vi "Get Channel Details.vi"(11 "Channel Parameters In":T1={"Channel Name"="0", "Number of Records"=0, "Reference Position"=0.0, "Minimum Record Length"=0, "Minimum Sample Rate"=0.0, "Maximum Input Frequency"=0.0, "Enforce Realtime"=FALSE, "Vertical Coupling"=enum."AC", "Probe Attenuation"=0.0, "Vertical Range (V)"=0.0, "Vertical Offset"=0.0, "Trigger Level"=0.0, "Trigger Type"=enum."Edge", "Trigger Source"=enum."Immediate", "Trigger Slope"=enum."Positive", "Digitizer 1 Used?"=FALSE, "Digitizer 1 Channels"="", "Digitizer 1 Reference"="", "Digitizer 1 Gain Multiplier"=nan, "Digitizer 2 Used?"=FALSE, "Digitizer 2 Channels"="", "Digitizer 2 Reference"="", "Session References"=[]}) -> (3 "Channel Parameters Out":T1={"Channel Name"="0", "Number of Records"=0, "Reference Position"=0.0, "Minimum Record Length"=0, "Minimum Sample Rate"=0.0, "Maximum Input Frequency"=0.0, "Enforce Realtime"=FALSE, "Vertical Coupling"=enum."AC", "Probe Attenuation"=0.0, "Vertical Range (V)"=0.0, "Vertical Offset"=0.0, "Trigger Level"=0.0, "Trigger Type"=enum."Edge", "Trigger Source"=enum."Immediate", "Trigger Slope"=enum."Positive", "Digitizer 1 Used?"=FALSE, "Digitizer 1 Channels"="", "Digitizer 1 Reference"="", "Digitizer 1 Gain Multiplier"=nan, "Digitizer 2 Used?"=FALSE, "Digitizer 2 Channels"="", "Digitizer 2 Reference"="", "Session References"=[]})   [LabVIEW 2010]
doc: "This function parses the \"Channel Name\" field into \"Digitizer 1 Channels\" and \"Digitizer 2 Channels\" fields.\n\nFrom the Channel Name (4 Channels) seperated by comma, extract two Channels each for the two Digitizers\n(a) Channel Name 1,2 Corresponds to Channel 0 and 1 of the first Digitizer\n(b) Channel Name 3,4 Corresponds to Channel 0 and 1 of the Second Digitizer"
uses:
  Typedef-Channel Parameters.ctl
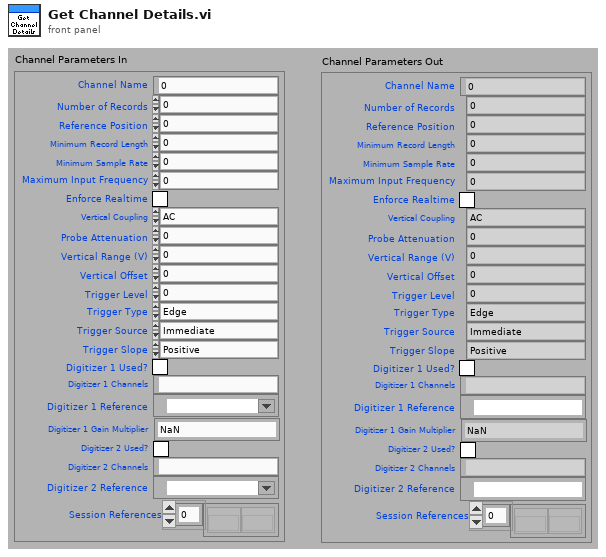
[diagram p1: front panel]
types:
  T1 = typedef "Typedef-Channel Parameters.ctl" = cluster{"Channel Name":string, "Number of Records":i32, "Reference Position":dbl, "Minimum Record Length":i32, "Minimum Sample Rate":dbl, "Maximum Input Frequency":dbl, "Enforce Realtime":bool, "Vertical Coupling":enum16{"AC", "DC", "Ground"}, "Probe Attenuation":dbl, "Vertical Range (V)":dbl, "Vertical Offset":dbl, "Trigger Level":dbl, "Trigger Type":enum16{"Edge", "Digital", "Immediate"}, "Trigger Source":enum16{"Immediate", "Channel 0", "Channel 1", "Channel 2", "Channel 3", "Channel 4", "Channel 5", "Channel 6", "Channel 7", "Extermal TRIG", "Software Trigger", "RTSI 0", "RTSI 1", "RTSI 2", "RTSI 3", "RTSI 4", "RTSI 5", "RTSI 6", "PF 0", "PF 1", "PF 2", "PXI Star Trigger"}, "Trigger Slope":enum16{"Positive", "Negative"}, "Digitizer 1 Used?":bool, "Digitizer 1 Channels":string, "Digitizer 1 Reference":refnum<k15>, "Digitizer 1 Gain Multiplier":dbl, "Digitizer 2 Used?":bool, "Digitizer 2 Channels":string, "Digitizer 2 Reference":refnum<k15>, "Session References":refnum<k20>[]}
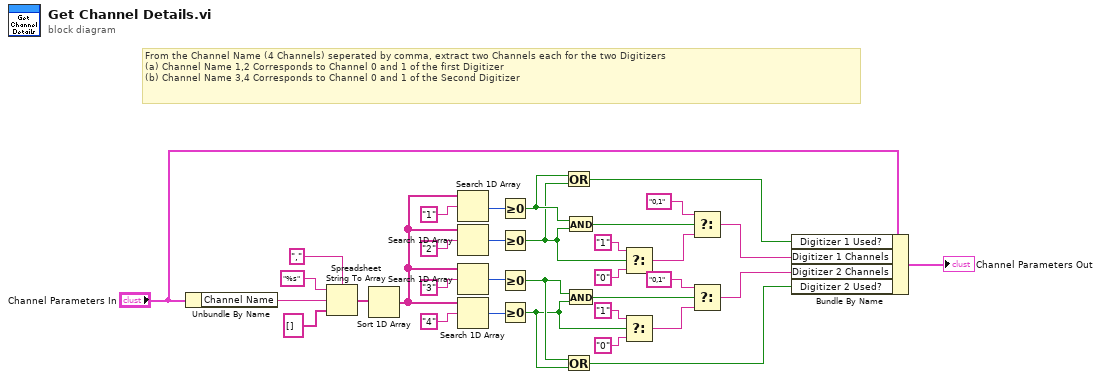
[diagram p0: block diagram]
diagram:
  # "From the Channel Name (4 Channels) seperated by comma, extract two Channels each for the two Digitizers\n(a) Channel Name 1,2 Corresponds to Channel 0 and 1 of the first Digitizer\n(b) Channel Name 3,4 Corresponds to Channel 0 and 1 of the Second Digitizer"
  n1 = Unbundle By Name("Channel Parameters In") -> ("Channel Name"=w7:string)
  n2 = Spreadsheet String To Array(delimiter (Tab)=",", format string="%s", spreadsheet string=w7, array type (2D Dbl)=string[] []) -> (array=w32:string[])
  n3 = Sort 1D Array(array=w32) -> (sorted array=w31:string[])
  n4 = Search 1D Array(1D array=w31, element="1") -> (index of element=w26:i32)  [unwired: 1 in]
  n5 = Search 1D Array(1D array=w31, element="2") -> (index of element=w23:i32)  [unwired: 1 in]
  n6 = Search 1D Array(1D array=w31, element="3") -> (index of element=w24:i32)  [unwired: 1 in]
  n7 = Search 1D Array(1D array=w31, element="4") -> (index of element=w25:i32)  [unwired: 1 in]
  n8 = Greater Or Equal To 0?(x=w26) -> (x >= 0?=w22:bool)
  n9 = Greater Or Equal To 0?(x=w23) -> (x >= 0?=w18:bool)
  n10 = Greater Or Equal To 0?(x=w24) -> (x >= 0?=w21:bool)
  n11 = Greater Or Equal To 0?(x=w25) -> (x >= 0?=w9:bool)
  n12 = Or(x=w22, y=w18) -> (x .or. y?=w5:bool)
  n13 = Or(x=w21, y=w9) -> (x .or. y?=w2:bool)
  n14 = And(x=w22, y=w18) -> (x .and. y?=w20:bool)
  n15 = And(x=w21, y=w9) -> (x .and. y?=w10:bool)
  n16 = Select(t="1", s=w18, f="0") -> (s? t:f=w16:string)
  n17 = Select(t="1", s=w9, f="0") -> (s? t:f=w12:string)
  n18 = Select(t="0,1", s=w20, f=w16) -> (s? t:f=w4:string)
  n19 = Select(t="0,1", s=w10, f=w12) -> (s? t:f=w3:string)
  n20 = Bundle By Name(cluster="Channel Parameters In", "Digitizer 1 Used?"=w5, "Digitizer 1 Channels"=w4, "Digitizer 2 Channels"=w3, "Digitizer 2 Used?"=w2) -> (→"Channel Parameters Out":T1)
